vi "Set Board LED State.vi"(8 "error in (no error)":errorcluster, 10 "LED State":bool, 11 "GE 5565PIORC in":refnum<class "GE 5565PIORC.lvclass">) -> (0 "error out":errorcluster, 3 "GE 5565PIORC out":refnum<class "GE 5565PIORC.lvclass">)   [LabVIEW 2016, in "GE 5565PIORC.lvclass"]
uses:
  GE 5565PIORC.lvclass
  GE 5565PIORC.lvclass/GE 5565PIORC.ctl
  Binary Operations/Set Bits.vi
  Binary Operations/Set Bits U32.vi
  Registers/RFM Control and Status.Get Register Offset.vi
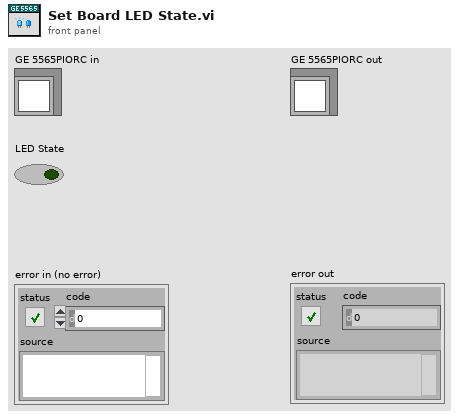
[diagram p1: front panel]
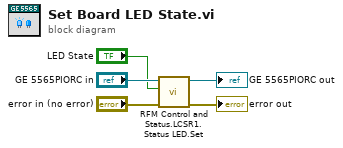
[diagram p0: block diagram]
diagram:
  n1 = call "RFM Control and Status.LCSR1.Status LED.Set.vi"("error in (no error)"="error in (no error)", "Status LED State"="LED State", "GE 5565PIORC"="GE 5565PIORC in") -> ("error out"=→"error out":errorcluster, "GE 5565PIORC out"=→"GE 5565PIORC out":refnum<class "GE 5565PIORC.lvclass">)  [unwired: 7 in]
